vi "JPL Joystick Select.vi"(0 "Joy 0 Axes":dbl[](array[numeric]), 1 "Joy 0 Left":dbl, 2 "Joy 0 Right":dbl, 5 "Joy 0 Buttons":bool[](array[boolean]), 9 "Joy 1 Axes":dbl[](array[numeric]), 11 "Joy 1 Buttons":bool[](array[boolean]), 12 "Joy 1 Left":dbl, 13 "Joy 1 Right":dbl, 14 "Servo Angle":dbl) -> (4 "Left Joy Out":dbl, 6 "Right Joy Out":dbl, 8 "Joy 0 Selected":bool, 10 "DS Axes Values":dbl[](array[numeric]), 15 "DS Buttons Values":bool[](array[boolean]))   [LabVIEW 2015]
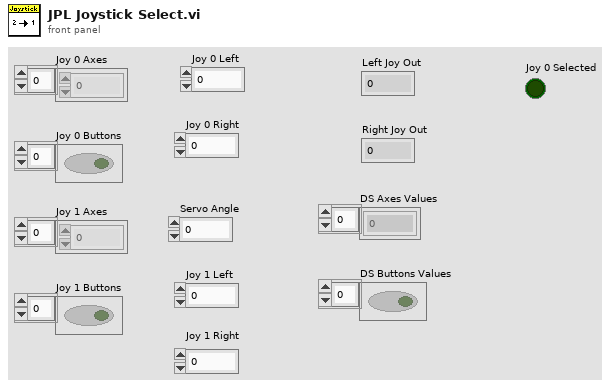
[diagram p1: front panel]
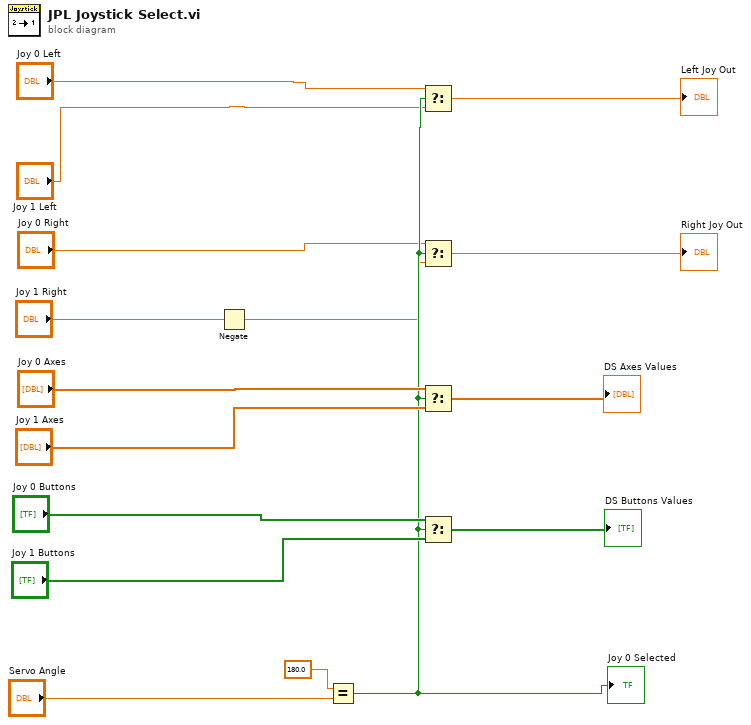
[diagram p0: block diagram]
diagram:
  n1 = Negate(x="Joy 1 Right") -> (-x=w3:dbl)
  n2 = Equal?(x=180.0, y="Servo Angle") -> (x = y?=w7:bool)
  "Joy 0 Selected" <- w7
  n3 = Select(t="Joy 0 Left", s=w7, f="Joy 1 Left") -> (s? t:f=→"Left Joy Out":dbl)
  n4 = Select(t="Joy 0 Right", s=w7, f=w3) -> (s? t:f=→"Right Joy Out":dbl)
  n5 = Select(t="Joy 0 Axes", s=w7, f="Joy 1 Axes") -> (s? t:f=→"DS Axes Values":dbl[])
  n6 = Select(t="Joy 0 Buttons", s=w7, f="Joy 1 Buttons") -> (s? t:f=→"DS Buttons Values":bool[])
